vi "Eval Parsed Formula String.vi"(2 "error in (no error)":errorcluster, 3 "Parsed Formula":cluster{"Table":i32[][], "Y Values":dbl[]} {"Y Values" format="%.2f"}, 4 "Variables":string[](array[string]), 5 "X Values":dbl[](array[numeric]) format="%0.2f") -> (0 "error out":errorcluster, 1 "y value":dbl format="%0.2f")   [LabVIEW 2020, in "NI_Gmath.lvlib"]
doc: "Takes the output of the Parse Formula String VI and fixes input values to calculate function values."
uses:
  NI_Gmath.lvlib
panel:
  # "Example:\n\n See Parse Formula String.vi!"
  # "operator"
  # "register1"
  # "register2"
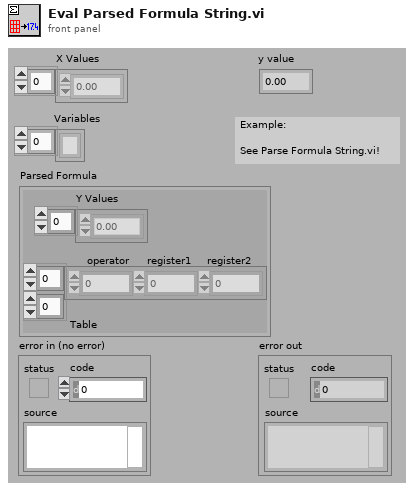
[diagram p1: front panel]
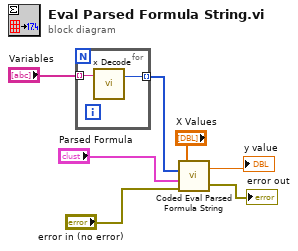
[diagram p0: block diagram]
diagram:
  n1 = for {
    tunnel: "Variables" -> [w9] mode=indexing
    tunnel: [w8] -> w4 mode=indexing
    n2 = call "x Decode.vi"("x string"=w9) -> ("number"=w8:i32)  [unwired: 1 in, 1 out]
  }
  n3 = call "Coded Eval Parsed Formula String.vi"("error in (no error)"="error in (no error)", "Parsed Formula"="Parsed Formula", "Variables"=w4, "X Values"="X Values") -> ("error out"=→"error out":errorcluster, "y value"=→"y value":dbl)
